vi "Approach then CV.vi"(7 "Computer called (T/F)":bool) -> ()   [LabVIEW 2023]
uses:
  Sub_Vi/TypeDefsControls/Zposition.ctl
  Sub_Vi/TypeDefsControls/Piezo Velocity.ctl
  Sub_Vi/TypeDefsControls/Voltage.ctl
  Sub_Vi/TypeDefsControls/Xposition.ctl
  Sub_Vi/TypeDefsControls/Yposition.ctl
  Sub_Vi/TypeDefsControls/Voltage Scan Rate.ctl
  Sub_Vi/TypeDefsControls/Iterator.ctl
  Sub_Vi/TypeDefs/WayPointCluster.ctl
  Sub_Vi/TypeDefs/ChangeOnFly.ctl
  Sub_Vi/TypeDefs/Settings.ctl
  Sub_Vi/TypeDefs/Display.ctl
  Sub_Vi/TypeDefsControls/Feedback Type.ctl
  Settings.vi
panel:
  in  "stop":bool
  in  "Feedback Type":T1
  in  "Tab Control":T2(tab)
  out "Current 1":cluster{"Y":dbl[], "Y":dbl[]}[](graph)
  out "Current 2":cluster{"Y":dbl[], "Y":dbl[]}[](graph)
  out "Current 3":cluster{"Y":dbl[], "Y":dbl[]}[](graph)
  in  "Display Cluster":T3
  in  "SettingsCluster":T4={"Sample Rate (us)"=1, "Samples Per Data Point (int, power of 2)"=1000, "DistanceToBulk (um)"=-1.0, "HoldTimeScaler"=1, "SaveData"=TRUE, "DistanceToBulk (um) 2"=-1.0, "DistanceToBulk (um) 3"=-1.0}
  in  "ChangeonFly":T5
  in  "WayPointCluster":T6
  in  "Number of Cycles":T7=1.0 min=1.0
  in  "Start scan Button":bool
  in  "Stop":bool
  in  "Pause":bool
  in  "Feedback Threshold (A)":dbl
  in  "Scan Rate (V/s)":T8 min=0.0 max=1000.0
  in  "Second Voltage (V)":T9 min=-10.0 max=10.0
  in  "First Voltage (V)":T9 min=-10.0 max=10.0
  in  "Greater Than":bool=TRUE
  in  "Set X":bool
  in  "Set Y":bool
  in  "Y":T10=50.0 min=0.0 max=100000.0
  in  "X":T11=50.0 min=0.0 max=100000.0
  in  "Approach Voltage (V)":T9=0.35 min=-10.0 max=10.0
  in  "Approach Rate (µm/s)":T12=0.1 min=0.0
  in  "End Extension (µm)":T13=38.0 min=0.0 max=100000.0
  in  "Start Extention (µm)":T13 min=0.0 max=100000.0
  out "C2 CV":cluster{"Y":dbl[], "Y":dbl[]}[](graph)
  out "C1 CV":cluster{"Y":dbl[], "Y":dbl[]}[](graph)
  in  "Start Scanning Button":bool
  out "Lock In Phase":dbl[](graph)
  out "Lock In Amplitude":dbl[](graph)
  # "Settings"
  # "Pause at"
  # "Advanced Settings"
  # "CV Controls"
  # "Voltage Profile"
  # "Approach"
  # "First Cycle"
  # "Additional Cycles"
  # "Retract"
  # "First\nVoltage"
  # "Approach\nVoltage"
  # "(Number of \ncycles)"
  # "Second\nVoltage"
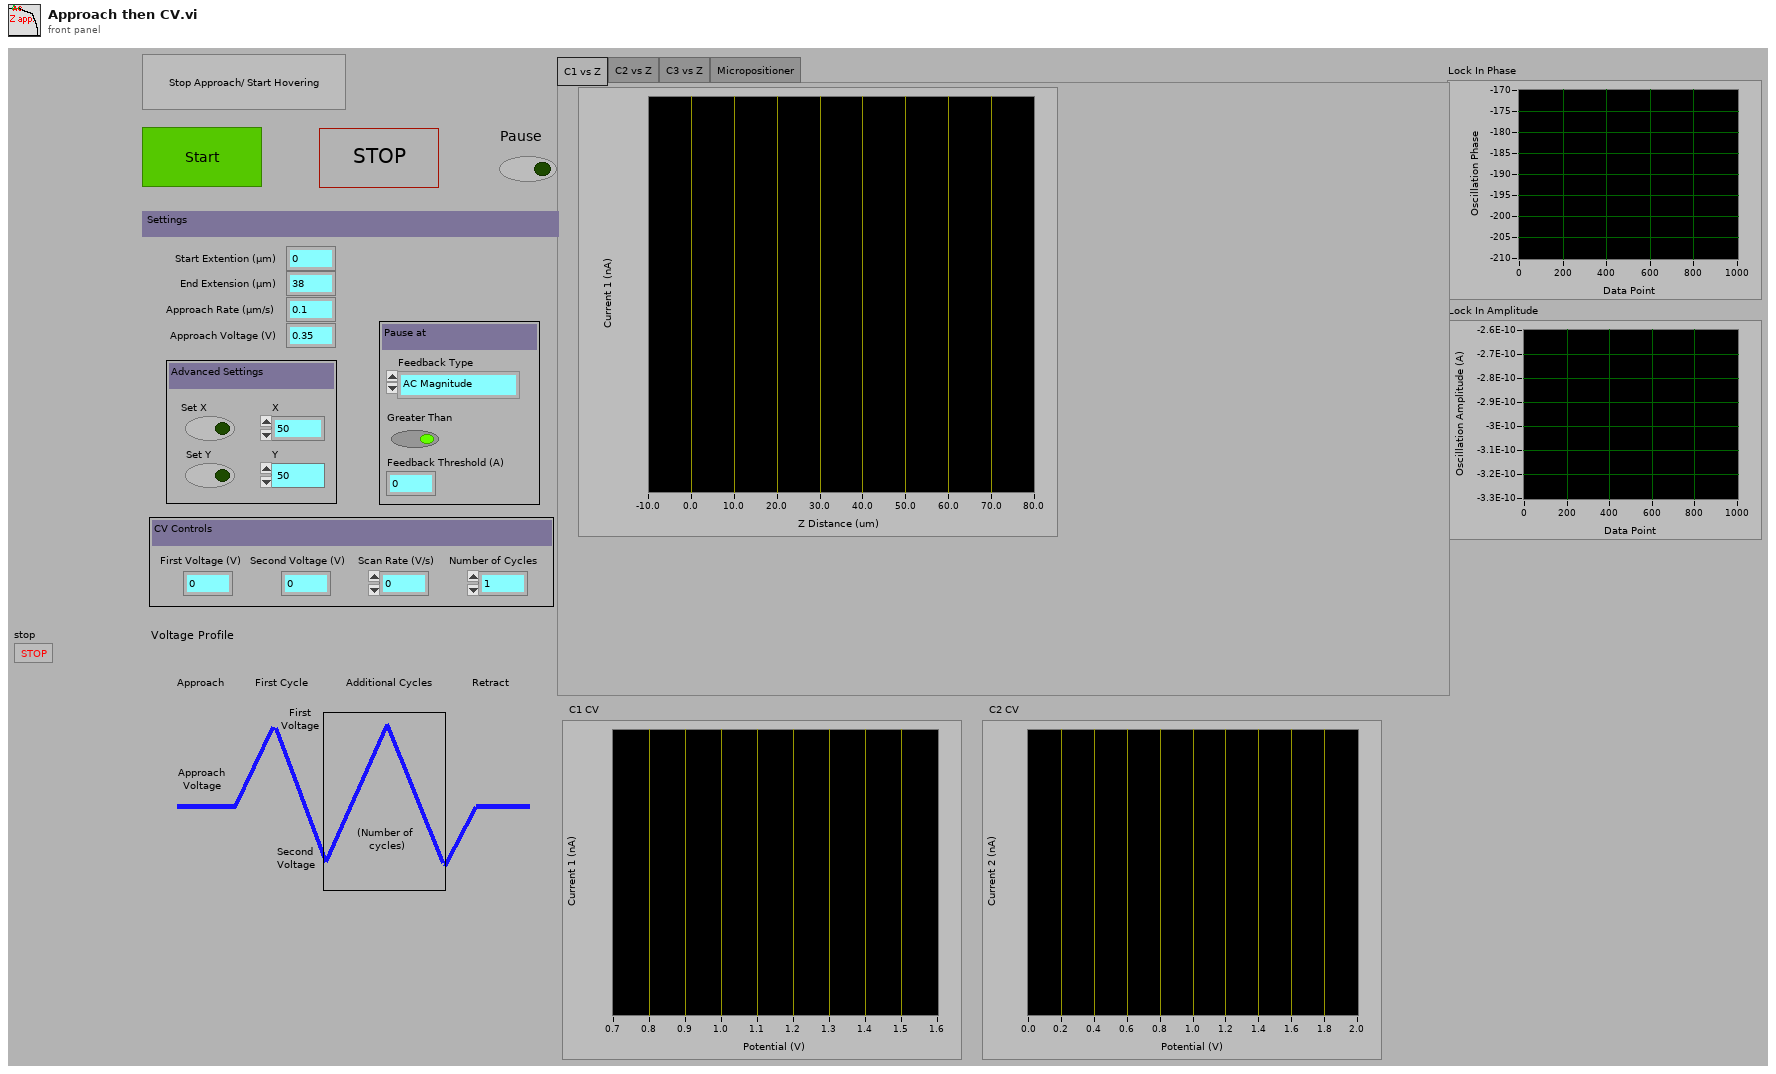
[diagram p1: front panel]
types:
  T1 = typedef "Feedback Type.ctl" = enum16{"AC Magnitude", "Current 1", "Current 2", "Phase"}
  T2 = enum32{"C1 vs Z", "C2 vs Z", "C3 vs Z", "Micropositioner"}
  T3 = typedef "Display.ctl" = cluster{"X":refnum<vi>, "Y":refnum<vi>, "Z":refnum<vi>, "Amp":refnum<vi>, "Phase":refnum<vi>, "t vs Z":refnum<vi>, "t vs C1":refnum<vi>, "t vs C2":refnum<vi>, "t vs C3":refnum<vi>, "t vs Amp":refnum<vi>, "t vs Phase":refnum<vi>, "t vs X":refnum<vi>, "t vs Y":refnum<vi>, "Z vs C1":refnum<vi>, "Z vs C2":refnum<vi>, "Z vs C3":refnum<vi>, "V vs C1":refnum<vi>, "V vs C2":refnum<vi>, "V vs C3":refnum<vi>, "X/Y/Z F":refnum<vi>, "X/Y/Z R":refnum<vi>, "X/Y/C1 F":refnum<vi>, "X/Y/C1 R":refnum<vi>, "X/Y/C2 F":refnum<vi>, "X/Y/C2 R":refnum<vi>, "X/Y/C3 F":refnum<vi>, "X/Y/C3 R":refnum<vi>, "NumberOfLines":u16, "um Per Pixel":dbl, "um Per Line":dbl, "X Center":dbl, "Hop X/Y/Z":refnum<vi>, "Hop X/Y/C1":refnum<vi>, "Hop X/Y/C2":refnum<vi>, "Hop X/Y/C3":refnum<vi>, "X Width":dbl, "Y Width":dbl, "Hopping Distance":dbl, "V2 vs C1":refnum<vi>, "V vs Phase":refnum<vi>, "Y Center":dbl, "Number of Pixels":dbl, "V2 vs C2":refnum<vi>, "V2 vs C3":refnum<vi>, "V vs y":refnum<vi>, "V2 vs y":refnum<vi>, "Z vs Amp":refnum<vi>, "Z vs Phase":refnum<vi>}
  T4 = typedef "Settings.ctl" = cluster{"Sample Rate (us)":u32, "Samples Per Data Point (int, power of 2)":i16, "DistanceToBulk (um)":dbl, "HoldTimeScaler":u64, "SaveData":bool, "DistanceToBulk (um) 2":dbl, "DistanceToBulk (um) 3":dbl}
  T5 = typedef "ChangeOnFly.ctl" = cluster{"Stop (boolean)":refnum<vi>, "Pause (boolean)":refnum<vi>, "EndCurrentLine (boolean)":refnum<vi>, "max movement per update step (Interger, nm)":refnum<vi>, "P (float, arb)":refnum<vi>, "Feedback set point (double, Amps)":refnum<vi>, "Voltage (double, V)":refnum<vi>, "Feedback set point 2 (double, Amps)":refnum<vi>, "Stop on Greater Than 2? (boolean)":refnum<vi>, "Stop on Greater Than? (boolean)":refnum<vi>, "Voltage 2 (double, V)":refnum<vi>, "Feedback Type (enum)":refnum<vi>, "Feedback Type 2 (enum)":refnum<vi>}
  T6 = typedef "WayPointCluster.ctl" = cluster{"X (um)":dbl[], "Y (um)":dbl[], "Z (um)":dbl[], "V (V)":dbl[], "X Velocity (um s-1)":dbl[], "Y Velocity (um s-1)":dbl[], "Z Velocity (um s-1)":dbl[], "V Velocity (V s-1)":dbl[], "FeedBack Type (enum)":u16[], "Move X (boolean)":bool[], "Move Y (boolean)":bool[], "Move Z (boolean)":bool[], "Move V (boolean)":bool[], "Jump V (boolean)":bool[], "Hold (boolean)":bool[], "Hold Time":u32[], "V2 (V)":dbl[], "Move V2":bool[], "V2 Velocity (V s-1)":dbl[], "Jump V2 (boolean)":bool[], "Update z Position delta (ms)":i16[], "Hold Feedback1":bool[], "Move Z PicoMotor":bool[], " Z PicoMotor Direction":bool[], "DIO0":bool[]}
  T7 = typedef "Iterator.ctl" = dbl
  T8 = typedef "Voltage Scan Rate.ctl" = dbl
  T9 = typedef "Voltage.ctl" = dbl
  T10 = typedef "Yposition.ctl" = dbl
  T11 = typedef "Xposition.ctl" = dbl
  T12 = typedef "Piezo Velocity.ctl" = dbl
  T13 = typedef "Zposition.ctl" = dbl
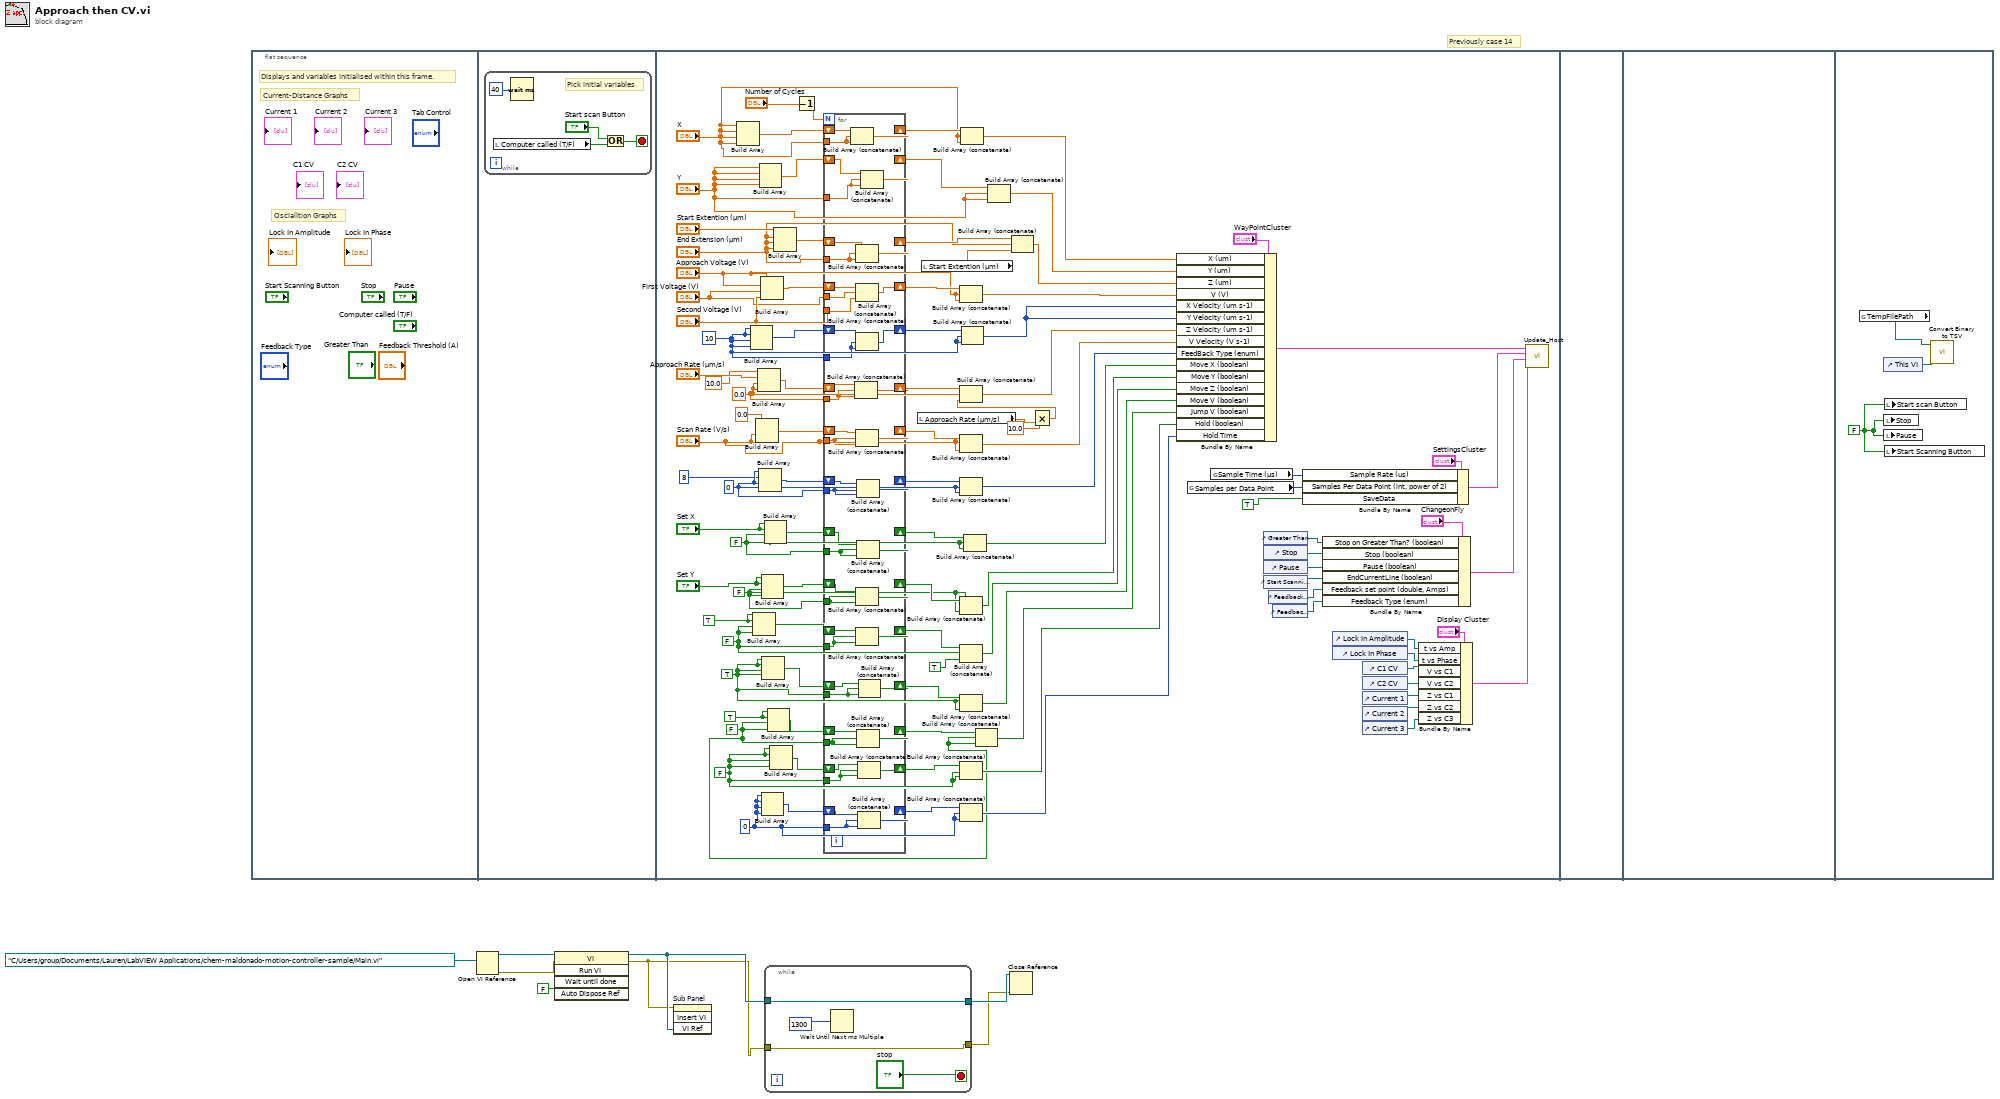
[diagram p0: block diagram]
diagram:
  # "Previously case 14"
  n1 = flat-sequence {
    frame #0 {
      # "Oscialltion Graphs"
      # "Current-Distance Graphs"
      # "Displays and variables initialised within this frame."
    }
    frame #1 {
      n2 = while {
        stop <- w12 stop-if-true
        # "Pick initial variables"
        n3 = local read "Computer called (T/F)"() -> (w10:bool)
        n4 = Wait (ms)(milliseconds to wait=u32 40) -> ()  [unwired: 1 out]
        n5 = Or(x="Start scan Button", y=w10) -> (x .or. y?=w12:bool)
      }
    }
    frame #2 {
      w16 = u32 0 ("element")
      w17 = FALSE ("element")
      w53 = TRUE ("Set Z")
      w19 = TRUE ("element")
      w91 = FALSE ("element")
      w22 = FALSE ("element")
      w21 = FALSE ("element")
      w23 = u16 0 ("element")
      w57 = 0.0
      w28 = 0.0 ("element")
      w18 = FALSE ("Set Z")
      w54 = TRUE ("Set Z")
      w29 = 10
      n6 = Build Array("X", "X", "X", "X") -> (w61:T11[])
      n7 = Build Array(w29, w29, w29, w29) -> (w76:i32[])
      n8 = Build Array(w54, w54, w91, w91) -> (w92:bool[])
      n9 = Build Array(w57, w57, "Scan Rate (V/s)", "Scan Rate (V/s)") -> (w81:T8[])
      n10 = Build Array(10.0 ("element"), "Approach Rate (µm/s)", w28, w28) -> (w79:T12[])
      n11 = Build Array(w23, u16 8 ("element"), w23, w23) -> (w84:u16[])
      n12 = Build Array("Y", "Y", "Y", "Y") -> (w64:T10[])
      n13 = Build Array("Approach Voltage (V)", "Approach Voltage (V)", "First Voltage (V)", "Second Voltage (V)") -> (w103:T9[])
      n14 = Build Array("Set Y", "Set Y", w21, w21) -> (w89:bool[])
      n15 = Build Array(w16, w16, w16, w16) -> (w102:u32[])
      n16 = Build Array(w19, w19, w19, w19) -> (w94:bool[])
      n17 = Build Array("Set X", "Set X", w22, w22) -> (w87:bool[])
      n18 = Build Array(w53, w53, w17, w17) -> (w96:bool[])
      n19 = Build Array(w18, w18, w18, w18) -> (w99:bool[])
      n20 = Build Array("Start Extention (µm)", "End Extension (µm)", "End Extension (µm)", "End Extension (µm)") -> (w38:T13[])
      n21 = Decrement(x="Number of Cycles") -> (x-1=w35:T7)
      n22 = for {
        N: w35 -> [_]
        tunnel: "First Voltage (V)" -> [w158]
        shift-right: [w159] -> w105
        shift-left: w103 -> [w160]
        tunnel: "Second Voltage (V)" -> [w157]
        shift-right: [w155] -> w101
        shift-left: w102 -> [w156]
        tunnel: w16 -> [w154]
        shift-right: [w151] -> w98
        shift-left: w99 -> [w152]
        tunnel: w18 -> [w153]
        shift-right: [w148] -> w95
        shift-left: w96 -> [w150]
        tunnel: w17 -> [w149]
        shift-right: [w146] -> w85
        shift-left: w94 -> [w147]
        tunnel: w19 -> [w145]
        shift-right: [w143] -> w93
        shift-left: w92 -> [w144]
        tunnel: w91 -> [w142]
        shift-right: [w140] -> w90
        shift-left: w89 -> [w141]
        tunnel: w21 -> [w139]
        shift-right: [w138] -> w86
        shift-left: w87 -> [w137]
        tunnel: w22 -> [w136]
        shift-right: [w134] -> w83
        shift-left: w84 -> [w135]
        tunnel: w23 -> [w133]
        shift-right: [w131] -> w82
        shift-left: w81 -> [w132]
        tunnel: "Scan Rate (V/s)" -> [w130]
        shift-right: [w128] -> w80
        shift-left: w79 -> [w129]
        tunnel: w28 -> [w127]
        shift-right: [w125] -> w77
        shift-left: w76 -> [w126]
        tunnel: w29 -> [w124]
        shift-right: [w123] -> w68
        shift-left: w38 -> [w122]
        tunnel: "End Extension (µm)" -> [w121]
        shift-right: [w119] -> w65
        shift-left: w64 -> [w120]
        tunnel: "Y" -> [w118]
        shift-right: [w116] -> w62
        shift-left: w61 -> [w117]
        tunnel: "X" -> [w115]
        n23 = Build Array (concatenate)(w117, w115, w115) -> (w116:T11[])
        n24 = Build Array (concatenate)(w129, w127, w127) -> (w128:T12[])
        n25 = Build Array (concatenate)(w122, w121, w121) -> (w123:T13[])
        n26 = Build Array (concatenate)(w160, w158, w157) -> (w159:T9[])
        n27 = Build Array (concatenate)(w126, w124, w124) -> (w125:i32[])
        n28 = Build Array (concatenate)(w141, w139, w139) -> (w140:bool[])
        n29 = Build Array (concatenate)(w132, w130, w130) -> (w131:T8[])
        n30 = Build Array (concatenate)(w144, w142, w142) -> (w143:bool[])
        n31 = Build Array (concatenate)(w135, w133, w133) -> (w134:u16[])
        n32 = Build Array (concatenate)(w137, w136, w136) -> (w138:bool[])
        n33 = Build Array (concatenate)(w150, w149, w149) -> (w148:bool[])
        n34 = Build Array (concatenate)(w152, w153, w153) -> (w151:bool[])
        n35 = Build Array (concatenate)(w156, w154, w154) -> (w155:u32[])
        n36 = Build Array (concatenate)(w147, w145, w145) -> (w146:bool[])
        n37 = Build Array (concatenate)(w120, w118, w118) -> (w119:T10[])
      }
      n38 = local read "Approach Rate (µm/s)"() -> (w27:T12)
      n39 = local read "Start Extention (µm)"() -> (w31:T13)
      n40 = Build Array (concatenate)(w105, "Approach Voltage (V)", "Approach Voltage (V)") -> (w104:T9[])
      n41 = Build Array (concatenate)(w82, "Scan Rate (V/s)", "Scan Rate (V/s)") -> (w69:T8[])
      n42 = Build Array (concatenate)(w83, w23, w23) -> (w70:u16[])
      n43 = Build Array (concatenate)(w90, w21, w21) -> (w71:bool[])
      n44 = Build Array (concatenate)(w93, w91, TRUE ("Set Z")) -> (w72:bool[])
      n45 = Build Array (concatenate)(w85, w19, w19) -> (w73:bool[])
      n46 = Build Array (concatenate)(w98, w18, w18) -> (w97:bool[])
      n47 = Build Array (concatenate)(w101, w16, w16) -> (w100:u32[])
      n48 = Build Array (concatenate)(w62, "X", "X") -> (w60:T11[])
      n49 = Build Array (concatenate)(w77, w29, w29) -> (w75:i32[])
      n50 = Build Array (concatenate)(w86, w22, w22) -> (w88:bool[])
      n51 = Build Array (concatenate)(w95, w17, w17) -> (w74:bool[])
      n52 = Build Array (concatenate)(w65, "Y", "Y") -> (w63:T10[])
      n53 = Build Array (concatenate)(w68, "End Extension (µm)", w31) -> (w66:T13[])
      n54 = Multiply(x=T12 10.0, y=w27) -> (x*y=w25:T12)
      n55 = Build Array (concatenate)(w80, w28, w25) -> (w78:T12[])
      n56 = Bundle By Name(cluster="WayPointCluster", "X (um)"=w60, "Y (um)"=w63, "Z (um)"=w66, "V (V)"=w104, "X Velocity (um s-1)"=w75, "Y Velocity (um s-1)"=w75, "Z Velocity (um s-1)"=w78, "V Velocity (V s-1)"=w69, "FeedBack Type (enum)"=w70, "Move X (boolean)"=w88, "Move Y (boolean)"=w71, "Move Z (boolean)"=w72, "Move V (boolean)"=w73, "Jump V (boolean)"=w74, "Hold (boolean)"=w97, "Hold Time"=w100) -> (w114:T6)
      n57 = global read "Settings.vi" "Samples per Data Point"() -> (w49:u16)
      n58 = global read "Settings.vi" "Sample Time (µs)"() -> (w50:u32)
      n59 = control-ref of="Greater Than"() -> (w47:refnum<vi>)
      n60 = control-ref of="Stop"() -> (w108:refnum<vi>)
      n61 = control-ref of="Pause"() -> (w107:refnum<vi>)
      n62 = control-ref of="Start Scanning Button"() -> (w110:refnum<vi>)
      n63 = control-ref of="Feedback Threshold (A)"() -> (w39:refnum<vi>)
      n64 = control-ref of="Feedback Type"() -> (w40:refnum<vi>)
      n65 = Bundle By Name(cluster="SettingsCluster", "Sample Rate (us)"=w50, "Samples Per Data Point (int, power of 2)"=w49, "SaveData"=TRUE) -> (w112:T4)
      n66 = Bundle By Name(cluster="ChangeonFly", "Stop on Greater Than? (boolean)"=w47, "Stop (boolean)"=w108, "Pause (boolean)"=w107, "EndCurrentLine (boolean)"=w110, "Feedback set point (double, Amps)"=w39, "Feedback Type (enum)"=w40) -> (w111:T5)
      n67 = control-ref of="Lock In Amplitude"() -> (w106:refnum<vi>)
      n68 = control-ref of="Lock In Phase"() -> (w36:refnum<vi>)
      n69 = control-ref of="C1 CV"() -> (w46:refnum<vi>)
      n70 = control-ref of="C2 CV"() -> (w45:refnum<vi>)
      n71 = control-ref of="Current 1"() -> (w44:refnum<vi>)
      n72 = control-ref of="Current 2"() -> (w43:refnum<vi>)
      n73 = control-ref of="Current 3"() -> (w37:refnum<vi>)
      n74 = Bundle By Name(cluster="Display Cluster", "t vs Amp"=w106, "t vs Phase"=w36, "V vs C1"=w46, "V vs C2"=w45, "Z vs C1"=w44, "Z vs C2"=w43, "Z vs C3"=w37) -> (w113:T3)
      n75 = call "Update_Host.vi"("Display Cluster"=w113, "ChangeonFly"=w111, "SettingsCluster"=w112, "WayPointCluster"=w114) -> ()  [unwired: 6 in]
    }
    frame #3 {
    }
    frame #4 {
    }
    frame #5 {
      w162 = FALSE ("Start Scanning Button")
      n76 = global read "Settings.vi" "TempFilePath"() -> (w161:path)
      n77 = control-ref of="This VI"() -> (w163:refnum<vi>)
      n78 = local write "Stop"(w162) -> ()
      n79 = local write "Pause"(w162) -> ()
      n80 = local write "Start scan Button"(w162) -> ()
      n81 = local write "Start Scanning Button"(w162) -> ()
      n82 = call "Convert Binary to TSV.vi"("This VI"=w163, "TDMS DataFile Name"=w161) -> ()  [unwired: 10 in]
    }
  }
  n83 = Open VI Reference(vi path=path "C:/Users/group/Documents/Lauren/LabVIEW Applications/chem-maldonado-motion-controller-sample/Main.vi" ("vi path 2")) -> (vi reference=w7:refnum<vi>, error out=w2:errorcluster)  [unwired: 5 in]
  n84 = invoke class="VI" method="Run VI"(reference=w7, error in=w2, "Wait until done"=FALSE ("Wait Until Done")) -> (reference out=w5:refnum<vi>, error out=w1:errorcluster)  [unwired: 2 in, 3 out]
  n85 = invoke on="Sub Panel" class="SubPnl" method="Insert VI"(error in=w1, "VI Ref"=w5) -> ()  [unwired: 2 in, 4 out]
  n86 = while {
    tunnel: w5 -> [w165]
    tunnel: [w165] -> w4
    tunnel: w1 -> [w164]
    tunnel: [w164] -> w3
    stop <- "stop" stop-if-true
    n87 = Wait Until Next ms Multiple(millisecond multiple=1300) -> ()  [unwired: 1 out]
  }
  n88 = Close Reference(reference=w4, error in (no error)=w3) -> ()  [unwired: 1 out]
